vi "PlanManager.vi"() -> ()   [LabVIEW 2020]
doc: "Fonction :\n\nCe modèle peut être intégré très facilement à un subpannel à l'aide des fonctions de la palette Code Template >> Dynamic VI and Subpanel de la VIBOX"
uses:
  <vilib>/DataGrid for LabVIEW/source/DataTable/DataTable.lvclass
  C:/Program Files (x86)/National Instruments/LabVIEW 2020/examples/DataGrid for LabVIEW/DataGrid.lvlib
  <vilib>/DataGrid for LabVIEW/source/DataGridView/DataGridView.lvclass
  <vilib>/DataGrid for LabVIEW/source/Events/CellClick/CellClick.lvclass
  System.Windows.Forms
panel:
  out "更新绑定":refnum<user-event>
  in  "确定":bool
  in  "产品型号":enum16{"SL7202", "SL7204"}(ring) caption="Enum 3"
  in  "计划数量":string
  in  "生产编号":string
  in  "选项":T1(radio)
  out "Stop<user event>":refnum<user-event>
  in  "DataGrid":refnum<k24>(container)
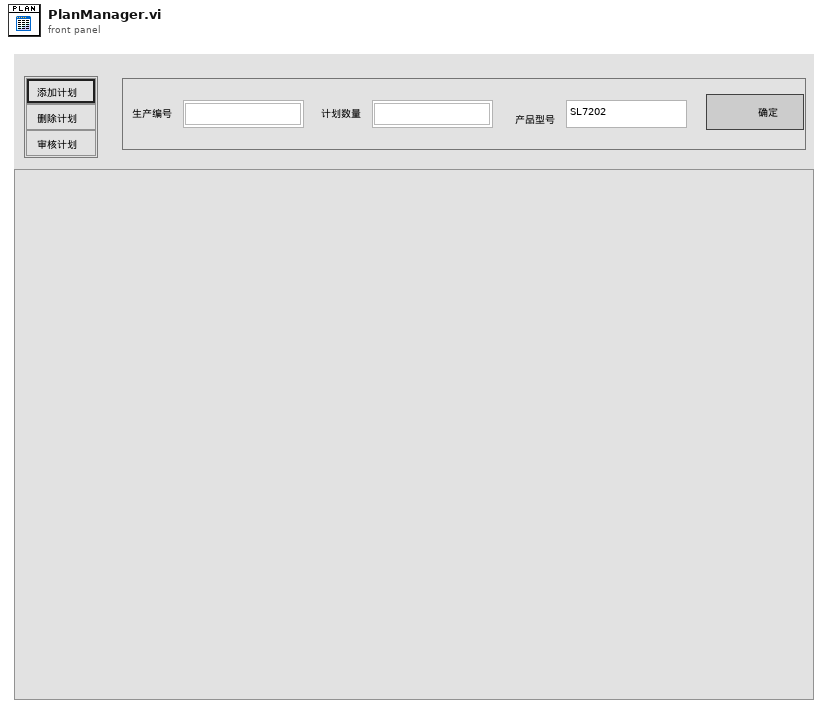
[diagram p1: front panel]
types:
  T1 = enum32{"Radio Selection 1", "Radio Selection 3", "Radio Selection 4"}
  T2 = typedef "DataGrid.lvlib/GridColumn.lvclass/ColumnDefinition.ctl" = cluster{"name":string, "caption":string, "datatype":T3, "Params":string, "AutoSizeMode":i32, "FillWeight":sgl, "MinWidth":u32, "tooltip":string}
  T3 = typedef "DataGrid.lvlib/GridColumn.lvclass/ColumnType.ctl" = enum16{"string", "image", "check", "numeric", "timestamp", "button", "combo", "link"}
  T4 = cluster{"CellClicked":refnum<user-event>, "CellValue Changed":refnum<user-event>, "KeyDown":refnum<user-event>, "DataError":refnum<user-event>, "UserAddedRow":refnum<user-event>, "UserDeletedRow":refnum<user-event>}
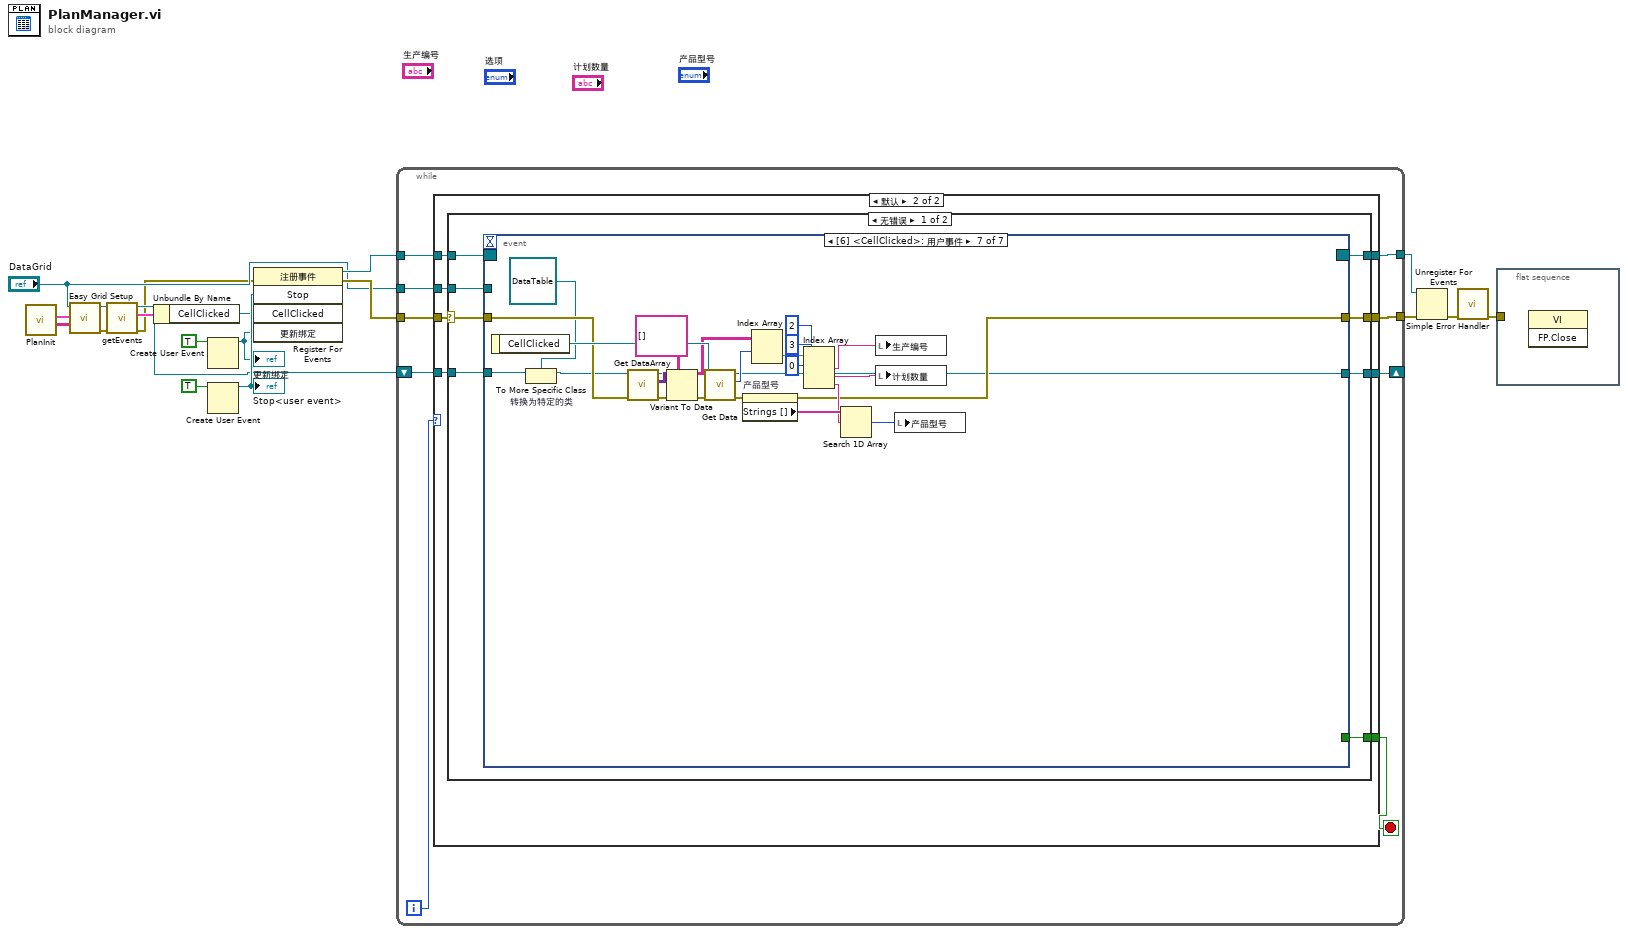
[diagram p0: block diagram]
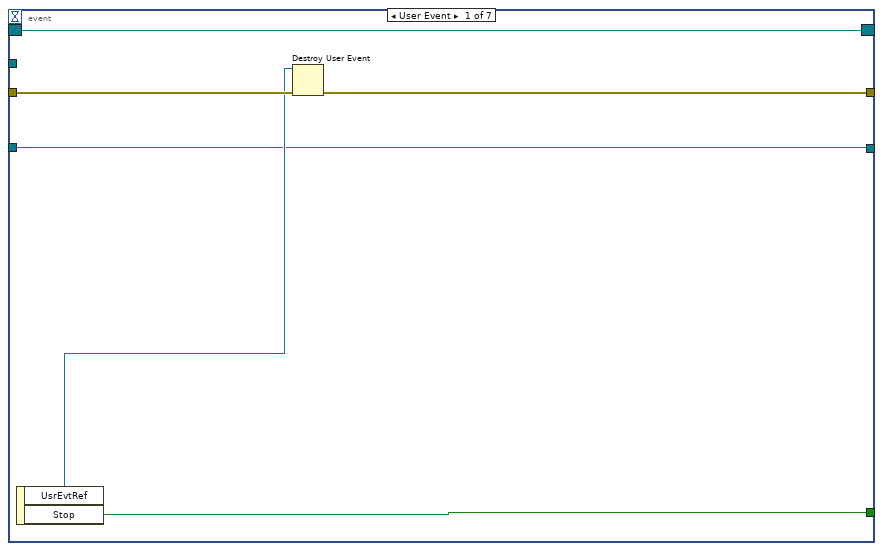
[diagram p3: hidden frame]
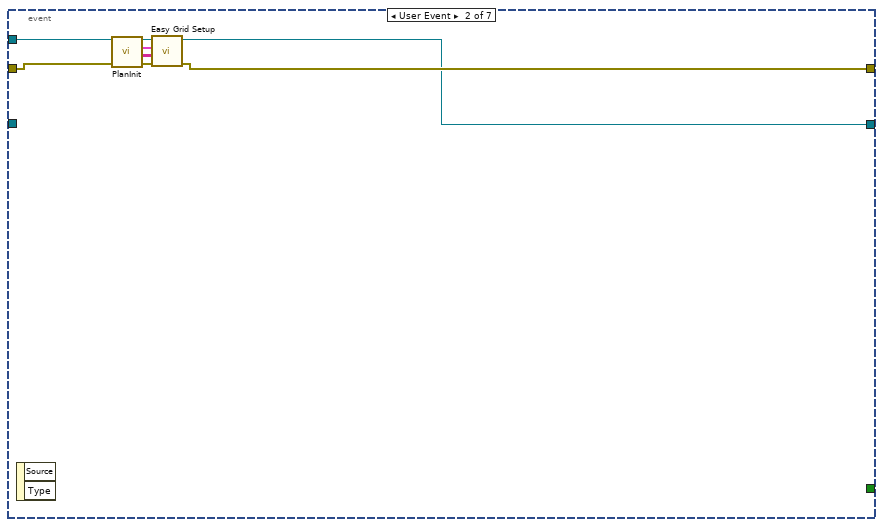
[diagram p4: hidden frame]
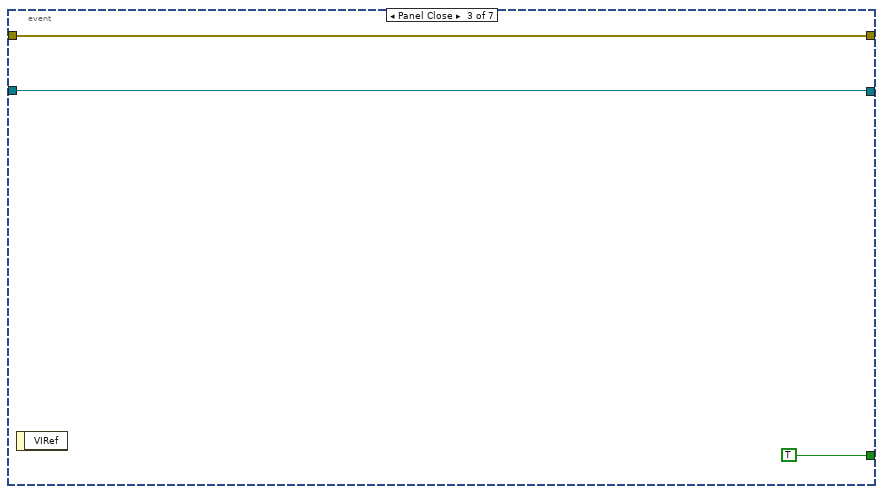
[diagram p5: hidden frame]
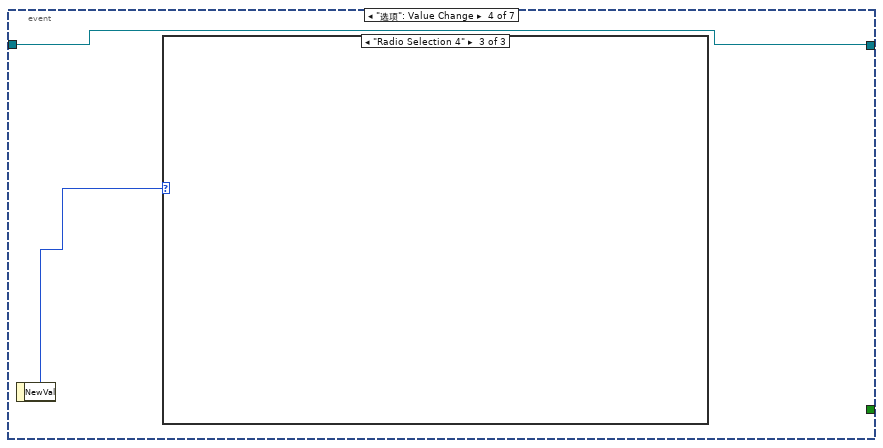
[diagram p6: hidden frame]
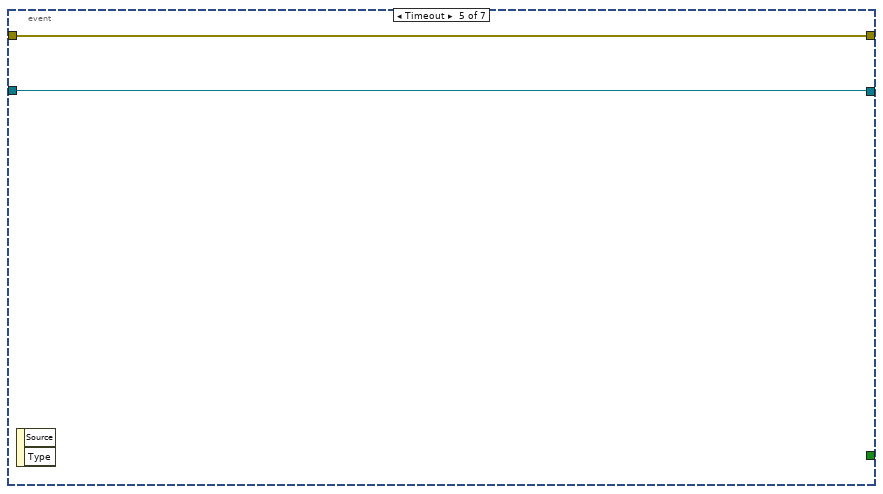
[diagram p9: hidden frame]
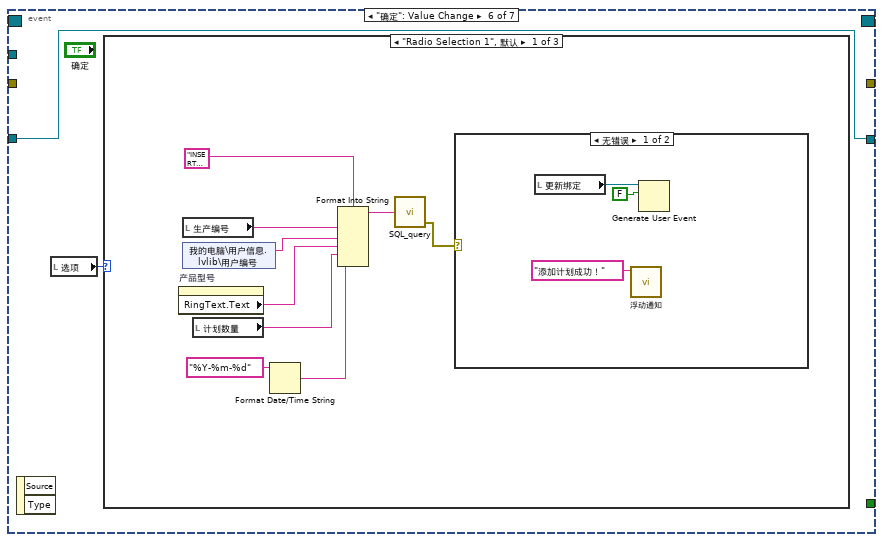
[diagram p10: hidden frame]
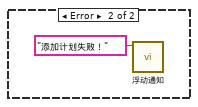
[diagram p11: hidden frame]
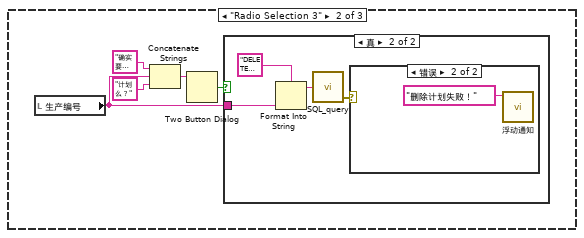
[diagram p12: hidden frame]
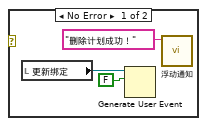
[diagram p14: hidden frame]
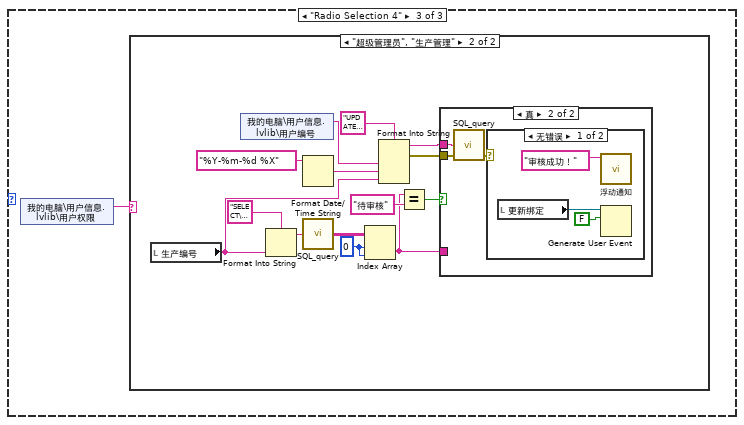
[diagram p15: hidden frame]
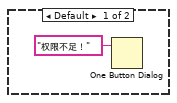
[diagram p16: hidden frame]
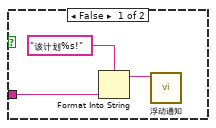
[diagram p17: hidden frame]
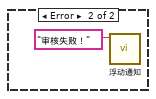
[diagram p18: hidden frame]
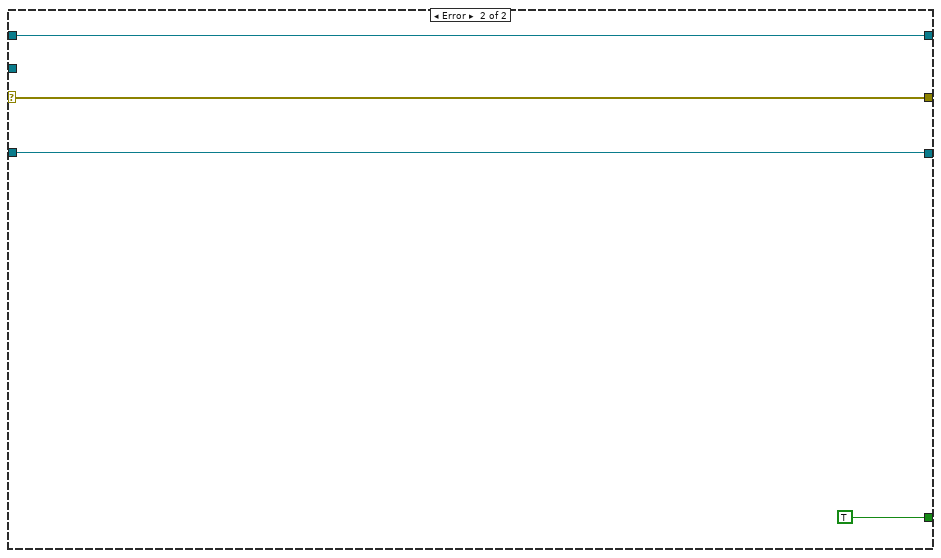
[diagram p19: hidden frame]
diagram:
  n1 = call "PlanInit.vi"() -> ("DataSource Data"=w2:string[][], "ColumnSetup"=w1:T2[])  [unwired: 10 in]
  n2 = call <vilib>:"Easy Grid Setup.vi"("DataSource Data"=w2, "ColumnSetup"=w1, "DataGridView"="DataGrid") -> ("error out"=w4:errorcluster, "DataGrid out"=w8:refnum<class "DataGridView.lvclass">)  [unwired: 5 in, 2 out]
  n3 = call <vilib>:"getEvents.vi"("error in (no error)"=w4, "DataGridView in"=w8) -> ("error out"=w3:errorcluster, "userEvents"=w7:T4, "DataGridView out"=w5:refnum<class "DataGridView.lvclass">)  [unwired: 7 in]
  n4 = Unbundle By Name(w7) -> ("CellClicked"=w6:refnum<user-event>)
  n5 = Create User Event(user event datatype=TRUE ("更新绑定")) -> (user event=w9:refnum<user-event>)  [unwired: 1 in, 1 out]
  "更新绑定" <- w9
  n6 = Create User Event(user event datatype=TRUE ("Stop")) -> (user event=w17:refnum<user-event>)  [unwired: 1 in, 1 out]
  "Stop<user event>" <- w17
  n7 = register-events(error in=w3, w17, w6, w9) -> (reference out=w16:refnum<event-registration>, error out=w12:errorcluster)  [unwired: 1 in]
  n8 = while {
    tunnel: w12 -> [w28]
    tunnel: [w27] -> w15
    tunnel: w16 -> [w25]
    tunnel: [w24] -> w19
    tunnel: "DataGrid" -> [w22]
    shift-right: [w20] -> _
    shift-left: w5 -> [w21]
    i -> [w23]
    stop <- w26 stop-if-true
    n9 = case shown="默认" w23 {
      tunnel: w28 -> [w30 w39]
      tunnel: [w30 w38] -> w27
      tunnel: [_ w37] -> w26
      tunnel: w25 -> [w31 w36]
      tunnel: [w31 w35] -> w24
      tunnel: w22 -> [_ w34]
      tunnel: w21 -> [w29 w33]
      tunnel: [w29 w32] -> w20
      frame 0 {
      }
      frame Default {
        n10 = case shown="无错误" w39 {
          selector: w39 -> [w44 w146]
          tunnel: [w43 w146] -> w38
          tunnel: [w45 TRUE] -> w37
          tunnel: w36 -> [w46 w145]
          tunnel: [w47 w145] -> w35
          tunnel: w34 -> [w42 _]
          tunnel: w33 -> [w41 w144]
          tunnel: [w40 w144] -> w32
          frame No Error {
            n11 = event shown="[6] <CellClicked>: 用户事件" {
              selector: w46 -> [w53 _ _ _ _ _ _]
              dyn-events: [w53 _ _ _ _ _ _] -> w47
              timeout: _ -> [_ _ _ _ _ _ _]
              tunnel: [w50 _ TRUE ("Stop") _ _ _ _] -> w45
              tunnel: w44 -> [w52 w59 w61 _ w66 _ w132]
              tunnel: [w49 w58 w61 _ w66 _ w128] -> w43
              tunnel: w42 -> [_ w57 _ _ _ _ _]
              tunnel: w41 -> [w48 _ w60 w63 w65 w67 w123]
              tunnel: [w48 w56 w60 w63 w65 w67 w127] -> w40
              event User Event {
                n12 = event-data() -> ("UsrEvtRef"=w51:refnum<user-event>, "Stop"=w50:bool)  [unwired: 1 out]
                n13 = Destroy User Event(user event=w51, error in=w52) -> (error out=w49:errorcluster)
              }
              event User Event {
                n14 = event-data() -> ()  [unwired: 3 out]
                n15 = call "PlanInit.vi"() -> ("DataSource Data"=w54:string[][], "ColumnSetup"=w55:T2[])  [unwired: 10 in]
                n16 = call <vilib>:"Easy Grid Setup.vi"("error in"=w59, "DataSource Data"=w54, "ColumnSetup"=w55, "DataGridView"=w57) -> ("error out"=w58:errorcluster, "DataGrid out"=w56:refnum<class "DataGridView.lvclass">)  [unwired: 4 in, 2 out]
              }
              event Panel Close {
                n17 = event-data() -> ()  [unwired: 2 out]
              }
              event "选项": Value Change {
                n18 = event-data() -> ("NewVal"=w64:T1)  [unwired: 1 out]
                n19 = case shown="\"Radio Selection 4\"" w64 {
                  frame "Radio Selection 1", Default {
                  }
                  frame "Radio Selection 3" {
                  }
                  frame "Radio Selection 4" {
                  }
                }
              }
              event Timeout {
                n20 = event-data() -> ()  [unwired: 3 out]
              }
              event "确定": Value Change {
                n21 = event-data() -> ()  [unwired: 3 out]
                n22 = local read "选项"() -> (w68:T1)
                n23 = case shown="\"Radio Selection 1\", 默认" w68 {
                  frame "Radio Selection 1", Default {
                    n24 = property on="产品型号" class="Enum (严格)"() -> ("RingText.Text"=w73:string)  [unwired: 2 in, 2 out]
                    n25 = local read "生产编号"() -> (w75:string)
                    n26 = shared-variable "我的电脑\\用户信息.lvlib\\用户编号"() -> (w74:string)  [unwired: 1 in, 1 out]
                    n27 = local read "计划数量"() -> (w72:string)
                    n28 = Format Date/Time String(time format string (%c)="%Y-%m-%d" ("时间格式字符串(%c)")) -> (date/time string=w71:string)  [unwired: 2 in]
                    n29 = Format Into String(format string="INSERT INTO [SanliServer].[dbo].[生产计划] ([生产编号], [操作员], [产品型号], [计划产量], [计划状态], [日期]) VALUES (N'%s', N'%s', N'%s', '%s', N'待审核', '%s')", w75, w74, w73, w72, w71) -> (resulting string=w77:string)  [unwired: 2 in, 1 out]
                    n30 = call "SQL_query.vi"("SQL query"=w77) -> ("error out"=w70:errorcluster)  [unwired: 3 in, 1 out]
                    n31 = case shown="无错误" w70 {
                      frame No Error {
                        n32 = local read "更新绑定"() -> (w79:refnum<user-event>)
                        n33 = call "浮动通知.vi"("通知内容"="添加计划成功！" ("消息")) -> ()  [unwired: 11 in]
                        n34 = Generate User Event(user event=w79, event data cluster=FALSE ("事件数据")) -> ()  [unwired: 2 in, 2 out]
                      }
                      frame Error {
                        n35 = call "浮动通知.vi"("通知内容"="添加计划失败！" ("消息")) -> ()  [unwired: 11 in]
                      }
                    }
                  }
                  frame "Radio Selection 3" {
                    n36 = local read "生产编号"() -> (w83:string)
                    n37 = Concatenate Strings("确实要删除", w83, "计划么？" ("字符串")) -> (w84:string)
                    n38 = Two Button Dialog(message=w84) -> (T button?=w82:bool)  [unwired: 2 in]
                    n39 = case shown="真" w82 {
                      tunnel: w83 -> [_ w87]
                      frame False {
                      }
                      frame True {
                        n40 = Format Into String(format string="DELETE FROM [SanliServer].[dbo].[生产计划] WHERE ([生产编号]=N'%s')", w87) -> (resulting string=w90:string)  [unwired: 2 in, 1 out]
                        n41 = call "SQL_query.vi"("SQL query"=w90) -> ("error out"=w89:errorcluster)  [unwired: 3 in, 1 out]
                        n42 = case shown="错误" w89 {
                          frame No Error {
                            n43 = local read "更新绑定"() -> (w92:refnum<user-event>)
                            n44 = Generate User Event(user event=w92, event data cluster=FALSE ("事件数据")) -> ()  [unwired: 2 in, 2 out]
                            n45 = call "浮动通知.vi"("通知内容"="删除计划成功！" ("消息")) -> ()  [unwired: 11 in]
                          }
                          frame Error {
                            n46 = call "浮动通知.vi"("通知内容"="删除计划失败！" ("消息")) -> ()  [unwired: 11 in]
                          }
                        }
                      }
                    }
                  }
                  frame "Radio Selection 4" {
                    n47 = shared-variable "我的电脑\\用户信息.lvlib\\用户权限"() -> (w95:string)  [unwired: 1 in, 1 out]
                    n48 = case shown="\"超级管理员\", \"生产管理\"" w95 {
                      frame Default {
                        n49 = One Button Dialog(message="权限不足！" ("消息")) -> ()  [unwired: 1 in, 1 out]
                      }
                      frame "超级管理员", "生产管理" {
                        w101 = 0 ("索引 (行)")
                        n50 = local read "生产编号"() -> (w97:string)
                        n51 = shared-variable "我的电脑\\用户信息.lvlib\\用户编号"() -> (w104:string)  [unwired: 1 in, 1 out]
                        n52 = Format Into String(format string="SELECT\ndbo.[生产计划].[计划状态]\nFROM\ndbo.[生产计划]\nWHERE\ndbo.[生产计划].[生产编号] = N'%s'", w97) -> (resulting string=w103:string)  [unwired: 2 in, 1 out]
                        n53 = Format Date/Time String(time format string (%c)="%Y-%m-%d %X" ("时间格式字符串(%c)")) -> (date/time string=w108:string)  [unwired: 2 in]
                        n54 = call "SQL_query.vi"("SQL query"=w103) -> ("data"=w102:string[][])  [unwired: 3 in, 1 out]
                        n55 = Index Array(array=w102, index (row)=w101, index (col)=w101) -> (element=w98:string)
                        n56 = Format Into String(format string="UPDATE [SanliServer].[dbo].[生产计划] SET [审核]=N'%s',\n[计划状态]=N'已审核', [审核时间]='%s' WHERE ([生产编号]=N'%s')", w104, w108, w97) -> (resulting string=w106:string, error out=w107:errorcluster)  [unwired: 2 in]
                        n57 = Equal?(x=w98, y="待审核") -> (x = y?=w99:bool)
                        n58 = case shown="真" w99 {
                          tunnel: w107 -> [_ w116]
                          tunnel: w106 -> [_ w115]
                          tunnel: w98 -> [w112 _]
                          frame False {
                            n59 = Format Into String(format string="该计划%s!" ("消息"), w112) -> (resulting string=w111:string)  [unwired: 2 in, 1 out]
                            n60 = call "浮动通知.vi"("通知内容"=w111) -> ()  [unwired: 11 in]
                          }
                          frame True {
                            n61 = call "SQL_query.vi"("error in (no error)"=w116, "SQL query"=w115) -> ("error out"=w114:errorcluster)  [unwired: 2 in, 1 out]
                            n62 = case shown="无错误" w114 {
                              frame No Error {
                                n63 = local read "更新绑定"() -> (w118:refnum<user-event>)
                                n64 = call "浮动通知.vi"("通知内容"="审核成功！" ("消息")) -> ()  [unwired: 11 in]
                                n65 = Generate User Event(user event=w118, event data cluster=FALSE ("事件数据")) -> ()  [unwired: 2 in, 2 out]
                              }
                              frame Error {
                                n66 = call "浮动通知.vi"("通知内容"="审核失败！" ("消息")) -> ()  [unwired: 11 in]
                              }
                            }
                          }
                        }
                      }
                    }
                  }
                }
              }
              event User Event {
                n67 = event-data() -> ("CellClicked"=w143:refnum<class "Abstract EVENT.lvclass">)  [unwired: 1 out]
                n68 = To More Specific Class "转换为特定的类"(target class=refnum<class "DataTable.lvclass"> refnum ("DataTable in"), reference=w123) -> (specific class reference=w121:refnum<class "DataTable.lvclass">)  [unwired: 1 in, 1 out]
                n69 = call <vilib>:"Get DataArray.vi"("error in (no error)"=w132, "DataTable in"=w121) -> ("error out"=w131:errorcluster, "Array"=w142:variant[][], "DataTable out"=w127:refnum<class "DataTable.lvclass">)  [unwired: 7 in]
                n70 = Variant To Data(error in=w131, type=string[][] [], Variant=w142) -> (data=w140:string[][], error out=w130:errorcluster)
                n71 = call <vilib>:"Get Data.vi"("error in (no error)"=w130, "DataGrid.lvlib:Abstract EVENT.lvclass"=w143) -> ("error out"=w129:errorcluster, "row"=w139:i32)  [unwired: 7 in, 1 out]
                n72 = property on="产品型号" class="Enum (严格)"(error in=w129) -> (error out=w128:errorcluster, "Strings []"=w135:string[])  [unwired: 1 in, 1 out]
                n73 = Index Array(array=w140, index (row)=w139) -> (element=w138:string[])  [unwired: 1 in]
                n74 = Index Array(array=w138, index #1=0 ("索引"), index #2=3 ("索引"), index #3=2 ("索引")) -> (element #1=w137:string, element #2=w136:string, element #3=w133:string)
                n75 = Search 1D Array(1D array=w135, element=w133) -> (index of element=w134:i32)  [unwired: 1 in]
                n76 = local write "生产编号"(w137) -> ()
                n77 = local write "计划数量"(w136) -> ()
                n78 = local write "产品型号"(w134) -> ()
              }
            }
          }
          frame Error {
          }
        }
      }
    }
  }
  n79 = Unregister For Events(event registration refnum=w19, error in=w15) -> (error out=w18:errorcluster)
  n80 = call <vilib>:"Simple Error Handler.vi"("error in (no error)"=w18) -> ("error out"=w13:errorcluster)  [unwired: 1 in, 7 out]
  n81 = flat-sequence {
    tunnel: w13 -> [_]
    frame #0 {
      n82 = invoke class="VI" method="FP.Close"() -> ()  [unwired: 3 in, 3 out]
    }
  }
